vi "assets.get.vi"(8 "error in (no error)":errorcluster, 11 "Run in":refnum<class "Run.lvclass">) -> (0 "error out":errorcluster, 2 "assets":string[](array[string]), 3 "Run out":refnum<class "Run.lvclass">)   [LabVIEW 2020, in "Run.lvclass"]
uses:
  Run.lvclass
  Run.lvclass/Run.ctl
  fc990382-c15b-405e-8523-435b97eca7cf.vi
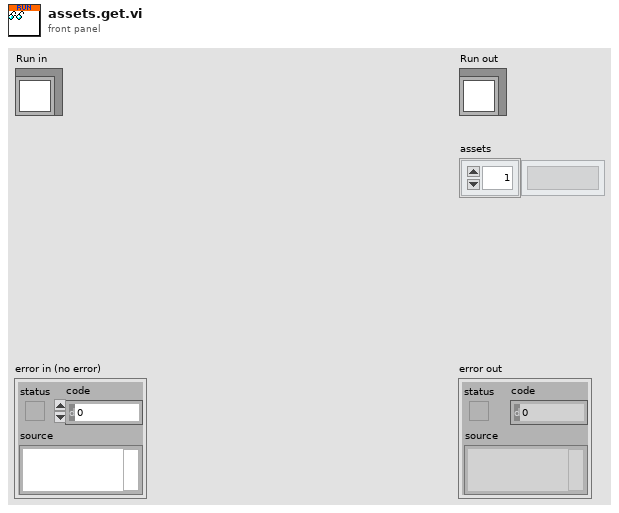
[diagram p1: front panel]
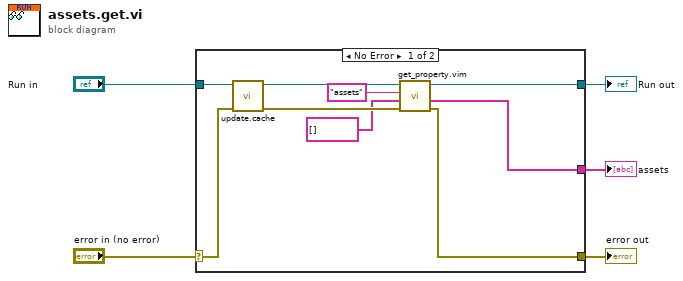
[diagram p0: block diagram]
diagram:
  n1 = case shown="No Error" "error in (no error)" {
    selector: "error in (no error)" -> [w14 w15]
    tunnel: [w7 w15] -> w4
    tunnel: [w8 w16] -> w2
    tunnel: "Run in" -> [w13 w16]
    tunnel: [w6 _] -> w1
    frame No Error {
      n2 = call "update.cache.vi"("error in"=w14, "Run in"=w13) -> ("error out"=w11:errorcluster, "Run out"=w12:refnum<class "Run.lvclass">)  [unwired: 8 in]
      n3 = call "get_property.vim"("error in"=w11, "default value and type"=string[] [] ("assets"), "Property Name"="assets", "Run in"=w12) -> ("error out"=w7:errorcluster, "Value"=w6:string[], "Run out"=w8:refnum<class "Run.lvclass">)  [unwired: 5 in]
    }
    frame Error {
    }
  }
  "error out" <- w4
  "Run out" <- w2
  "assets" <- w1
